vi "RT Loop - Analyze Acceleration.vi"(8 "error in (no error)":errorcluster, 9 "Acceleration RT FIFO In":T3, 10 "FPGA VI Reference Out":T2, 11 "Message Queue":refnum<queue>) -> (1 "Acceleration RT FIFO Out":T3)   [LabVIEW 2017]
doc: "Read and analyze acceleration waveform data from FPGA via DMA FIFO. If the acceleration is over the limit, then send the acceleration waveform data to the Log Data Loop."
uses:
  AI3568B Catapult 2017-18 top up/5 - Software Files/Sample Project/support/Message Queue/Message Cluster.ctl
  AI3568B Catapult 2017-18 top up/5 - Software Files/Sample Project/controls/Acceleration RT FIFO Reference.ctl
  AI3568B Catapult 2017-18 top up/5 - Software Files/Sample Project/FPGA Bitfiles/FPGA_ref.ctl
  AI3568B Catapult 2017-18 top up/5 - Software Files/Sample Project/Globals/Global - All RT Loop Stop.vi
  AI3568B Catapult 2017-18 top up/5 - Software Files/Sample Project/Globals/Global - Configuration Options.vi
  <vilib>/Utility/error.llb/Error Cluster From Error Code.vi
  <vilib>/rvi/errors/niLvFpgaAdjustHostInterfaceError.vi
  <vilib>/rvi/interface/nirviMethod/nirviMethod.xnode
  <vilib>/FPGAPlugInAG/Dynamic/niLvFpga_ReadFifo_Dynamic.vi
  <vilib>/rvi/errors/niLvFpgaMergeErrorWithErrorCode.vi
  AI3568B Catapult 2017-18 top up/5 - Software Files/Sample Project/support/Message Queue/Message Queue.lvlib
panel:
  out "Acceleration (grms) 2":waveform(dbl)[](graph)
  out "Acceleration (grms)":T1(graph)
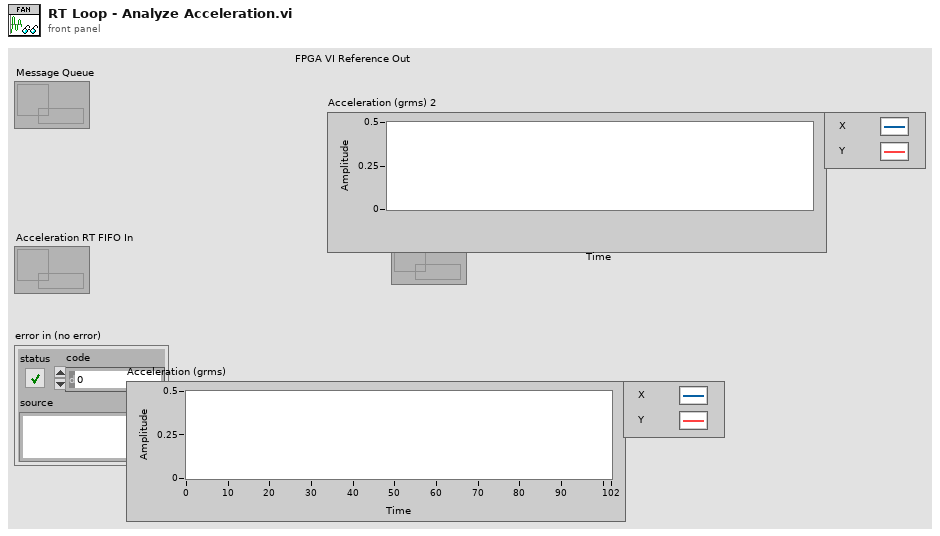
[diagram p1: front panel]
types:
  T1 = cluster{"Array of Double[0]":dbl, "Array of Double[1]":dbl}
  T2 = typedef "FPGA_ref.ctl" = refnum<k20>
  T3 = typedef "Acceleration RT FIFO Reference.ctl" = refnum<k33>
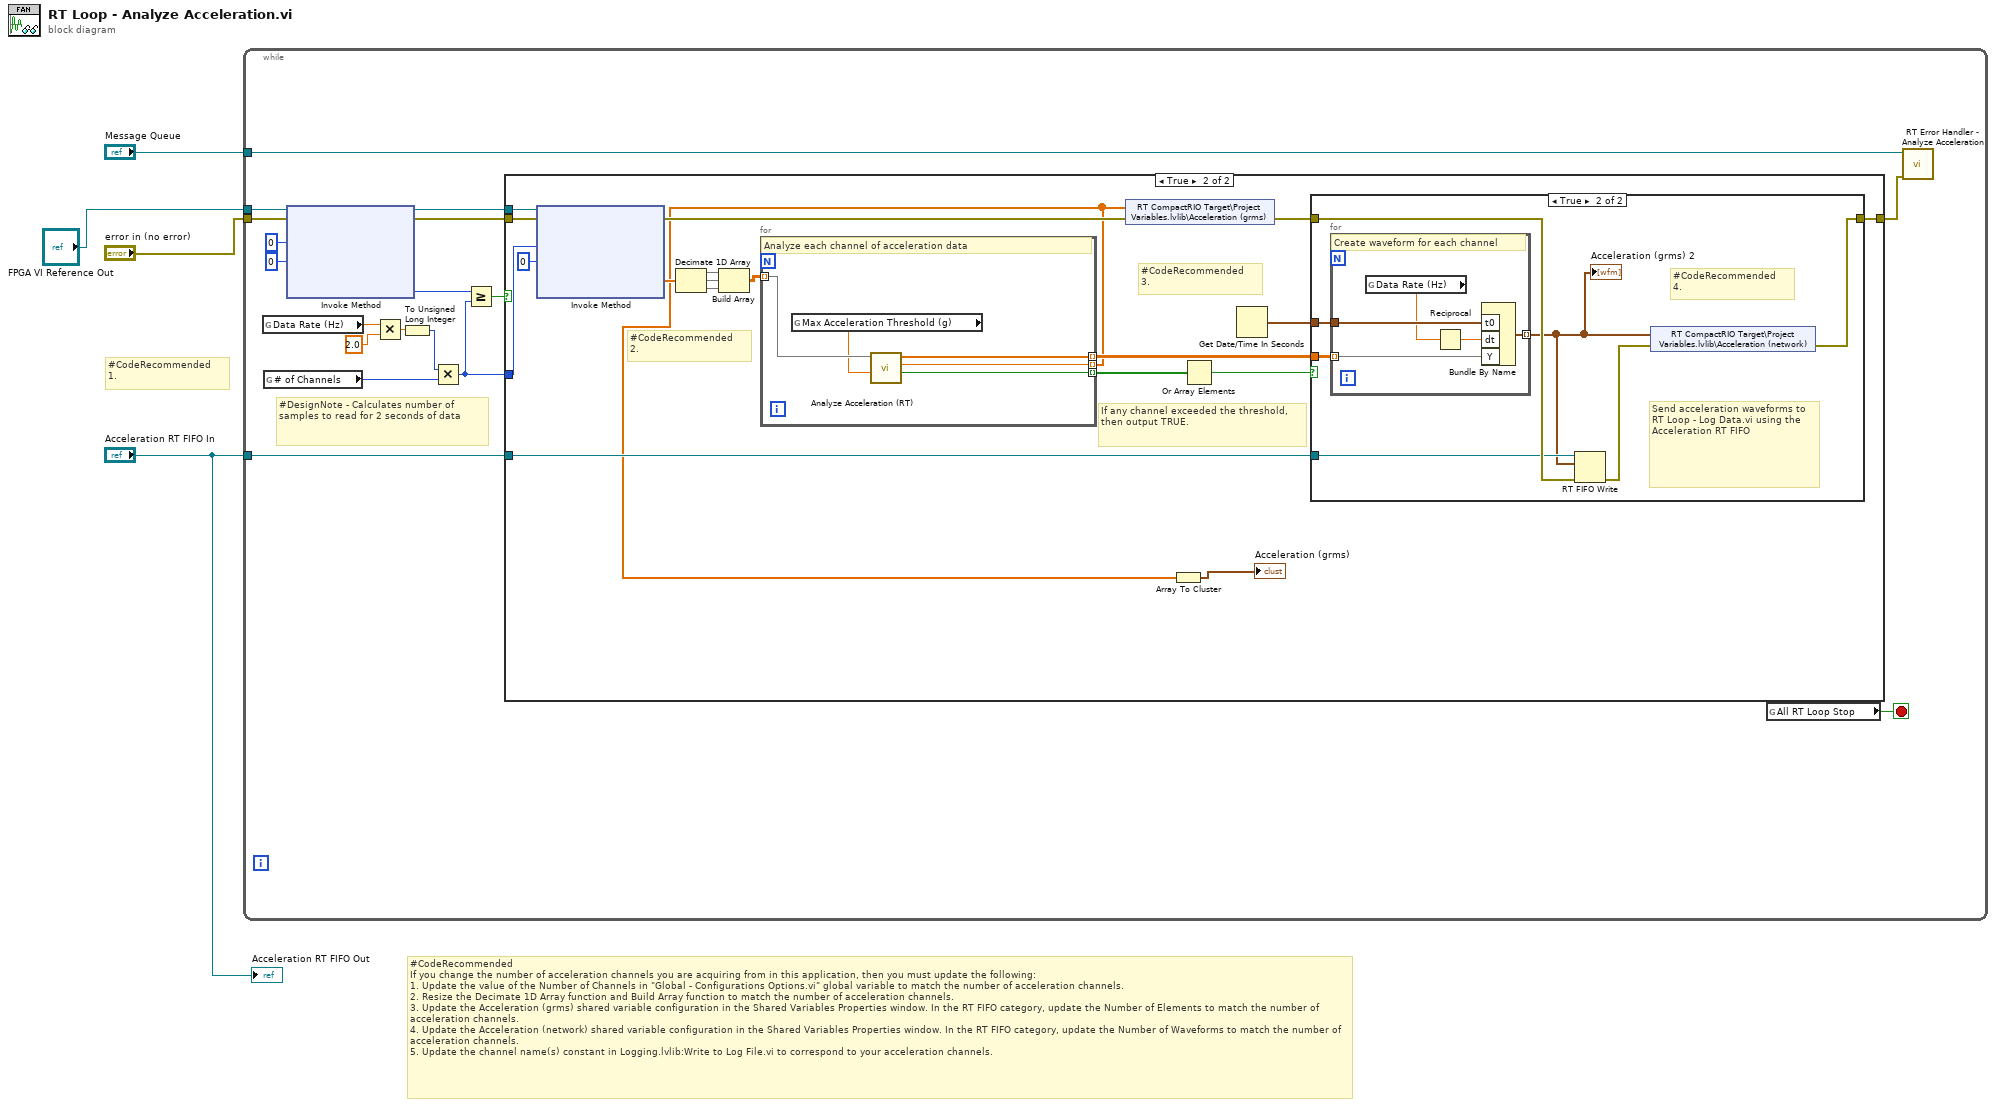
[diagram p0: block diagram]
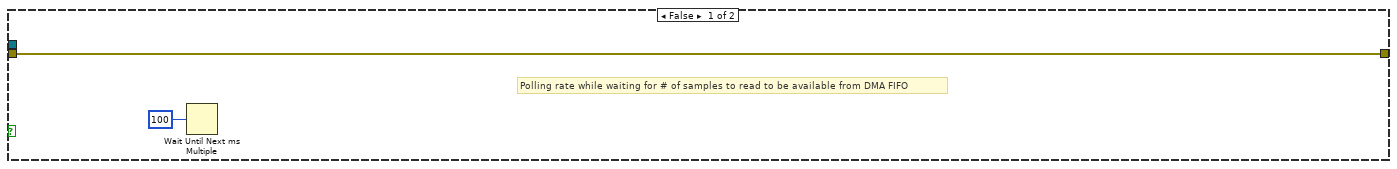
[diagram p2: hidden frame]
diagram:
  # "#CodeRecommended\n1."
  # "#CodeRecommended\nIf you change the number of acceleration channels you are acquiring from in this application, then you must update the following:\n1. Update the value of the Number of Channels in \"Global - Configurations Options.vi\" global variable to match the number of acceleration channels.\n2. Resize the Decimate 1D Array function and Build Array function to match the number of acceleration channels. \n3. Update the Acceleration (grms) shared variable configuration in the Shared Variables Properties window. In the RT FIFO category, update the Number of Elements to match the number of acceleration channels. \n4. Update the Acceleration (network) shared variable configuration in the Shared Variables Properties window. In the RT FIFO category, update the Number of Waveforms to match the number of acceleration channels.\n5. Update the channel name(s) constant in Logging.lvlib:Write to Log File.vi to correspond to your acceleration channels."
  n1 = while {
    tunnel: "FPGA VI Reference Out" -> [w22]
    tunnel: "error in (no error)" -> [w21]
    tunnel: "Message Queue" -> [w13]
    tunnel: "Acceleration RT FIFO In" -> [w11]
    stop <- w14 stop-if-true
    # "#DesignNote - Calculates number of samples to read for 2 seconds of data"
    n2 = global read "Global - Configuration Options.vi" "Data Rate (Hz)"() -> (w10:dbl)
    n3 = global read "Global - Configuration Options.vi" "# of Channels"() -> (w5:u32)
    n4 = xnode "Invoke Method"("FPGA VI Reference In"=w22, "error in"=w21, "Number of Elements"=u32 0, "Timeout (ms)"=0) -> ("FPGA VI Reference Out"=w17:T2, "error out"=w16:errorcluster, "Elements Remaining"=w18:u32)  [unwired: 1 out]
    n5 = Multiply(x=w10, y=2.0) -> (x*y=w8:dbl)
    n6 = To Unsigned Long Integer(number=w8) -> (unsigned 32bit integer=w7:u32)
    n7 = Multiply(x=w7, y=w5) -> (x*y=w6:u32)
    n8 = Greater Or Equal?(x=w18, y=w6) -> (x >= y?=w15:bool)
    n9 = case shown="True" w15 {
      tunnel: w17 -> [_ w43]
      tunnel: w16 -> [w24 w42]
      tunnel: [w24 w36] -> w12
      tunnel: w6 -> [_ w41]
      tunnel: w11 -> [_ w34]
      frame False {
        # "Polling rate while waiting for # of samples to read to be available from DMA FIFO"
        n10 = Wait Until Next ms Multiple(millisecond multiple=u32 100) -> ()  [unwired: 1 out]
      }
      frame True {
        # "If any channel exceeded the threshold, then output TRUE."
        # "#CodeRecommended\n3."
        # "#CodeRecommended\n2."
        n11 = xnode "Invoke Method"("FPGA VI Reference In"=w43, "error in"=w42, "Number of Elements"=w41, "Timeout (ms)"=0) -> ("error out"=w38:errorcluster, "Data"=w33:sgl[])  [unwired: 2 out]
        n12 = Decimate 1D Array(w33) -> (w32:sgl[], w31:sgl[], w25:sgl[])
        n13 = Build Array(w32, w31, w25) -> (w30:sgl[][])
        n14 = for {
          tunnel: [w48] -> w35 mode=indexing
          tunnel: [w47] -> w29 mode=indexing
          tunnel: [w46] -> w27 mode=indexing
          tunnel: w30 -> [w45] mode=indexing
          # "Analyze each channel of acceleration data"
          n15 = global read "Global - Configuration Options.vi" "Max Acceleration Threshold (g)"() -> (w44:sgl)
          n16 = call "Analyze Acceleration (RT).vi"("Max Instantaneous Acceleration (g)"=w44, "Acceleration Waveform (SGL)"=w45) -> ("Over Limit?"=w48:bool, "Acceleration (grms)"=w46:dbl, "Acceleration Waveform (DBL)"=w47:dbl[])  [unwired: 7 in]
        }
        n17 = shared-variable "RT CompactRIO Target\\Project Variables.lvlib\\Acceleration (grms)"(w27, error in=w38) -> (error out=w37:errorcluster)
        n18 = Array To Cluster(array=w27) -> (cluster=→"Acceleration (grms)":cluster{"[0]":dbl, "[1]":dbl})
        n19 = Or Array Elements(Boolean array=w35) -> (logical OR=w28:bool)
        n20 = Get Date/Time In Seconds() -> (seconds since 1Jan1904=w39:timestamp)
        n21 = case shown="True" w28 {
          tunnel: w39 -> [_ w56]
          tunnel: w37 -> [w49 w55]
          tunnel: [w49 w53] -> w36
          tunnel: w34 -> [_ w52]
          tunnel: w29 -> [_ w51]
          frame False {
          }
          frame True {
            # "#CodeRecommended\n4."
            # "Send acceleration waveforms to RT Loop - Log Data.vi using the Acceleration RT FIFO"
            n22 = for {
              tunnel: w51 -> [w61] mode=indexing
              tunnel: w56 -> [w60]
              tunnel: [w58] -> w50 mode=indexing
              # "Create waveform for each channel"
              n23 = global read "Global - Configuration Options.vi" "Data Rate (Hz)"() -> (w57:dbl)
              n24 = Reciprocal(x=w57) -> (1/x=w59:dbl)
              n25 = Bundle By Name("t0"=w60, "dt"=w59, "Y"=w61) -> (w58:waveform(dbl))  [unwired: 1 in]
            }
            "Acceleration (grms) 2" <- w50
            n26 = RT FIFO Write(0:w52, 1:w50, 3:w55) -> (11:w54:errorcluster)  [unwired: 2 in, 3 out]
            n27 = shared-variable "RT CompactRIO Target\\Project Variables.lvlib\\Acceleration (network)"(w50, error in=w54) -> (error out=w53:errorcluster)
          }
        }
      }
    }
    n28 = global read "Global - All RT Loop Stop.vi" "All RT Loop Stop"() -> (w14:bool)
    n29 = call "RT Error Handler - Analyze Acceleration.vi"("error in (no error)"=w12, "Message Queue"=w13) -> ()  [unwired: 9 in, 1 out]
  }
  "Acceleration RT FIFO Out" <- "Acceleration RT FIFO In"
